vi "MutiType to Enum.vi"(6 "Variant in":variant, 7 "Shift Pressed?":bool, 8 "error in (no error)":errorcluster, 10 "QD Combo Box Ref":refnum<vi>, 11 "QD Launch VI Ref":refnum<vi>) -> (0 "error out":errorcluster, 4 "Variant out":variant)   [LabVIEW 2017, in "String to Enum.lvlib"]
doc: "Converts the selected string, array, ring or combo box into an enum."
uses:
  String to Enum.lvlib
panel:
  in  "Undo Name":string="String to Enum"
  # "Do not change the connector pane of this VI.\n\nSee the block diagram for directions on how to use this template."
  # "Specify the name of the Undo transaction"
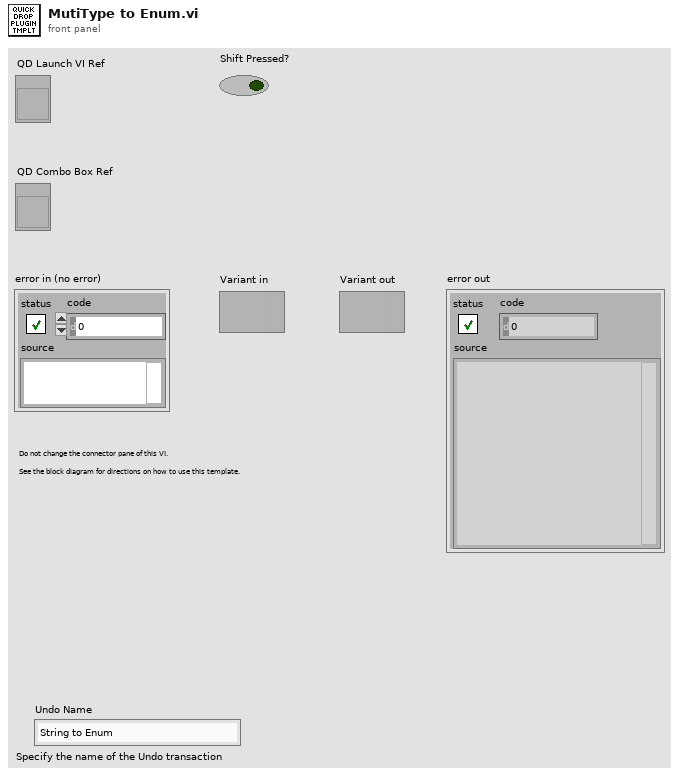
[diagram p1: front panel]
types:
  T1 = typedef "LVPositionTypeDef.ctl" = cluster{"Left":i32, "Top":i32}
  T2 = typedef "LVBoundsTypeDef.ctl" = cluster{"Width":u32, "Height":u32}
  T3 = typedef "LVComboBoxStrsAndValuesArrayTypeDef.ctl" = cluster{"String":string, "Value":string}[]
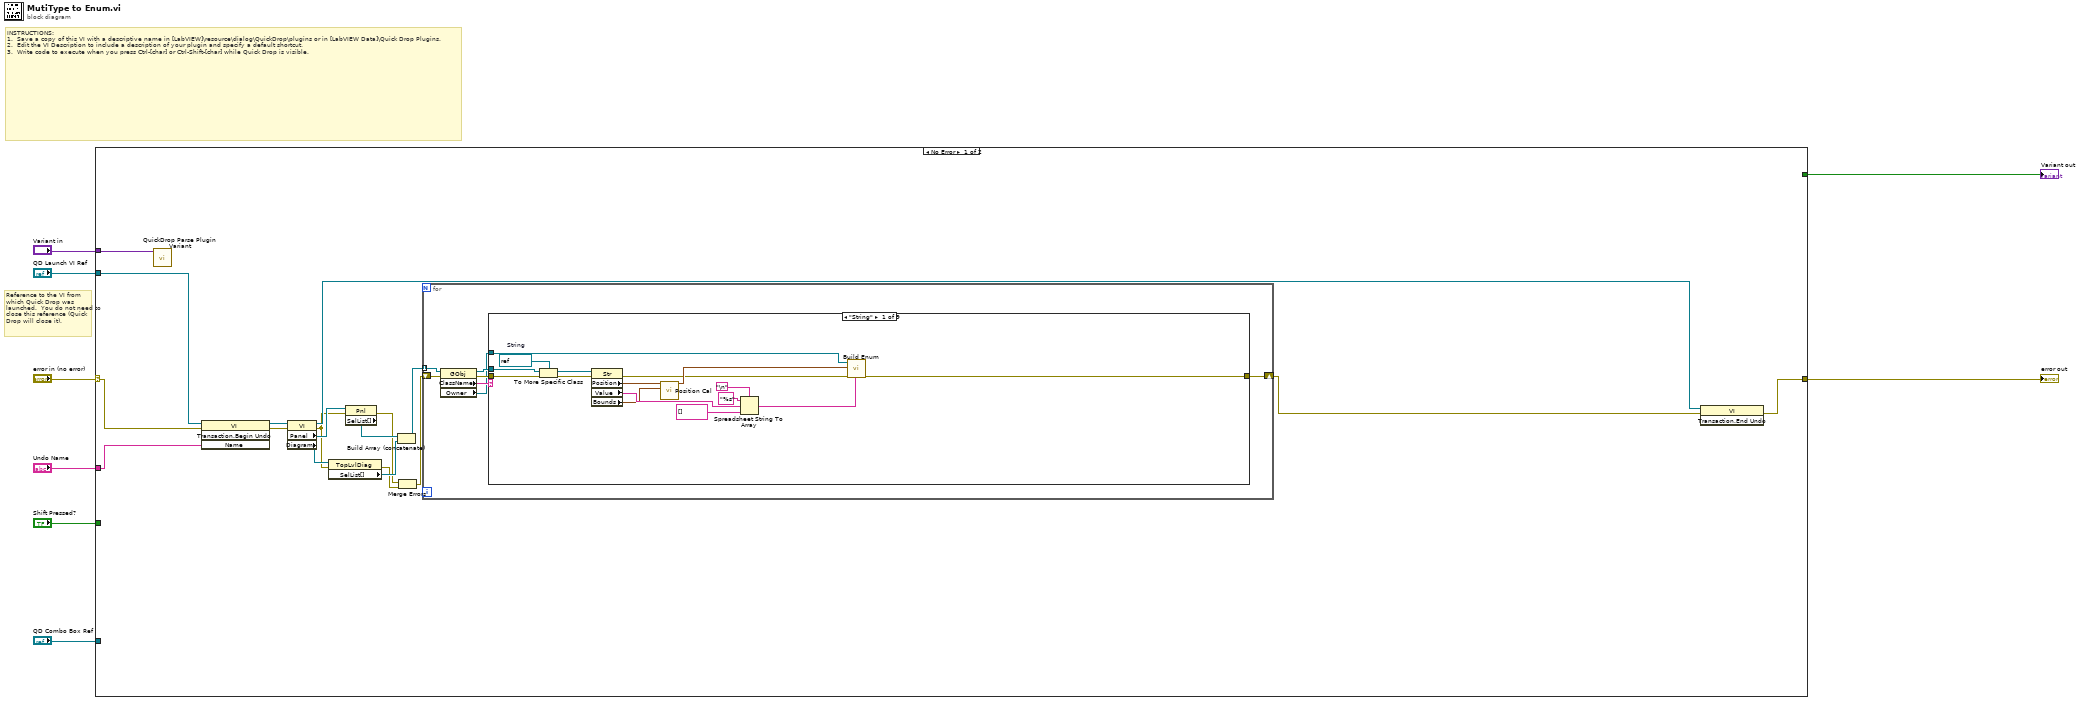
[diagram p0: block diagram]
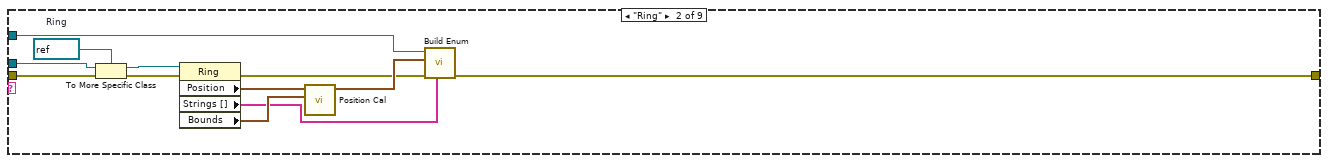
[diagram p2: hidden frame]
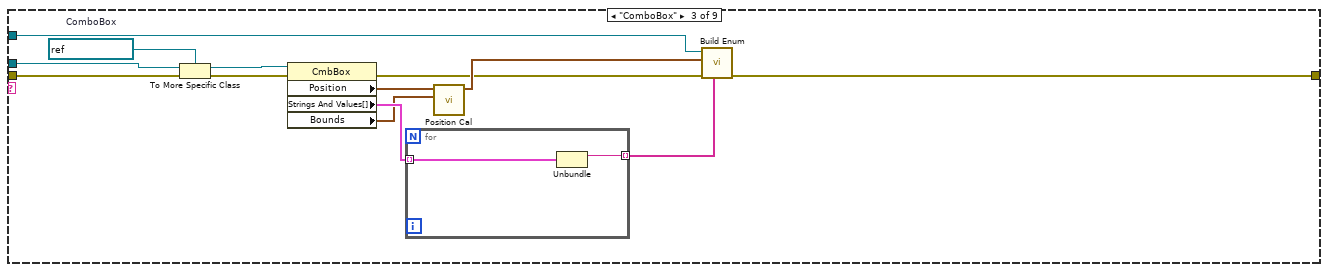
[diagram p3: hidden frame]
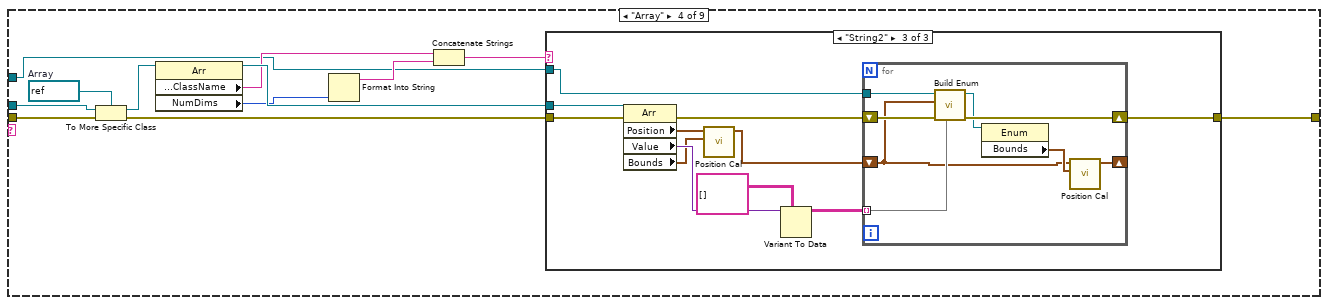
[diagram p4: hidden frame]
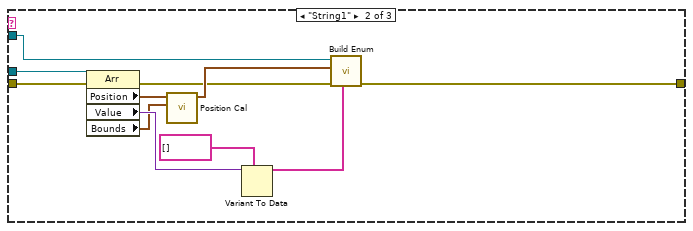
[diagram p6: hidden frame]
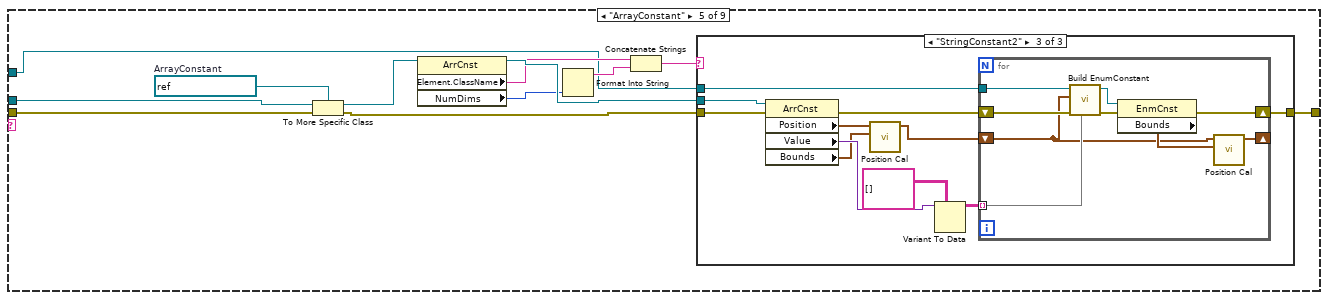
[diagram p7: hidden frame]
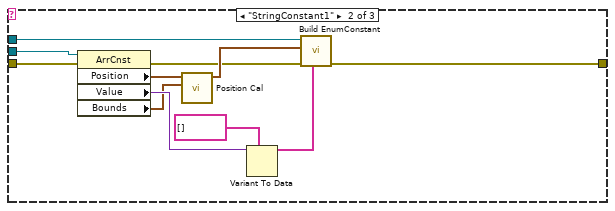
[diagram p9: hidden frame]
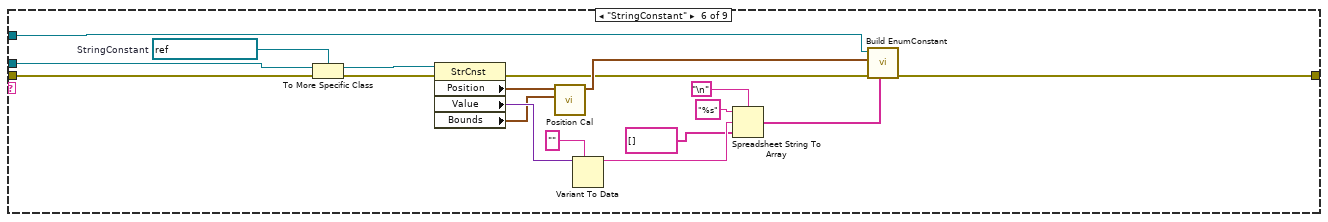
[diagram p10: hidden frame]
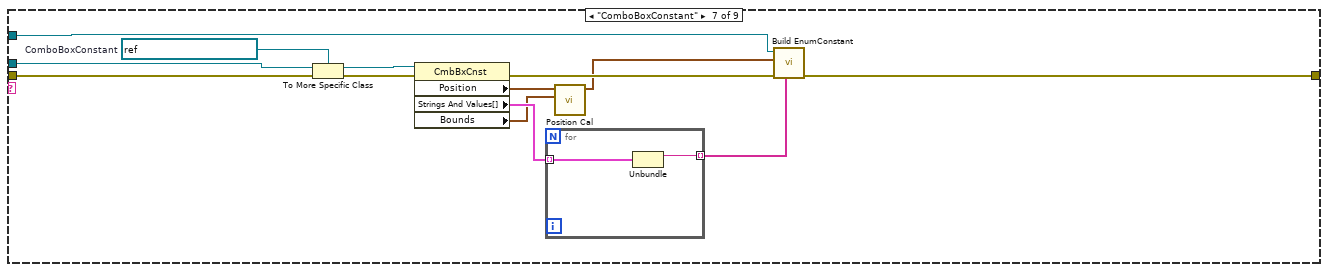
[diagram p11: hidden frame]
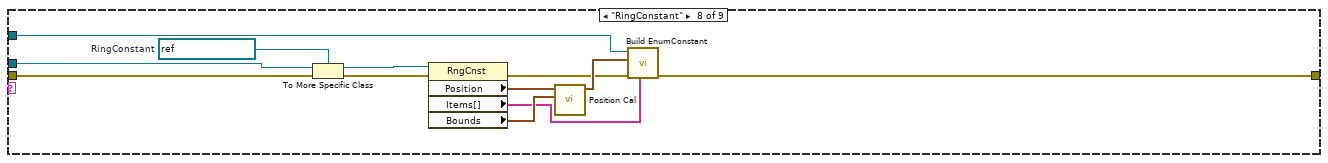
[diagram p12: hidden frame]
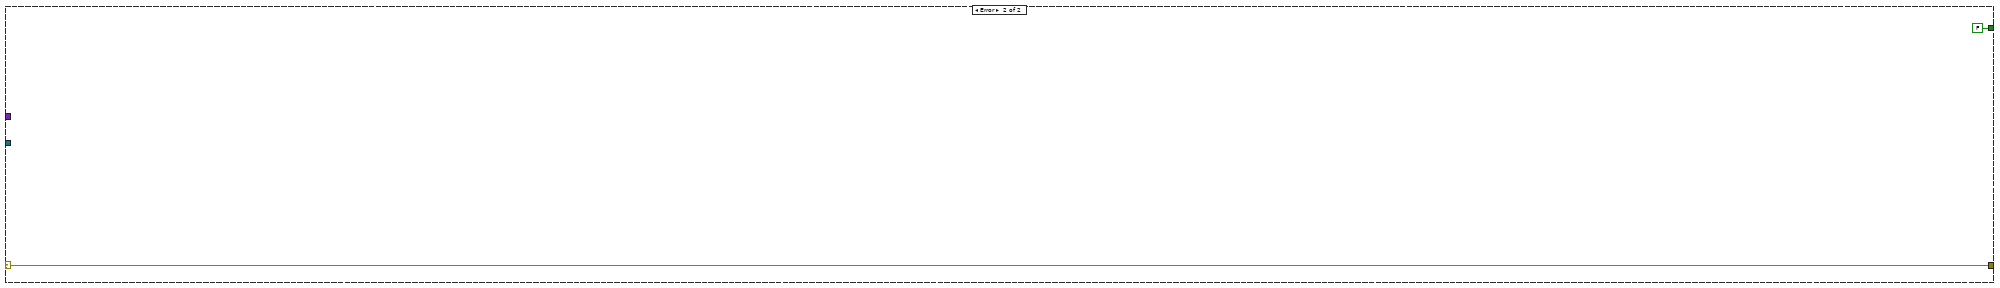
[diagram p14: hidden frame]
diagram:
  # "Reference to the VI from which Quick Drop was launched.  You do not need to close this reference (Quick Drop will close it)."
  # "INSTRUCTIONS:\n1.  Save a copy of this VI with a descriptive name in [LabVIEW]\\resource\\dialog\\QuickDrop\\plugins or in [LabVIEW Data]\\Quick Drop Plugins.\n2.  Edit the VI Description to include a description of your plugin and specify a default shortcut. \n3.  Write code to execute when you press Ctrl-[char] or Ctrl-Shift-[char] while Quick Drop is visible."
  n1 = case shown="No Error" "error in (no error)" {
    selector: "error in (no error)" -> [w23 w211]
    tunnel: [w20 w211] -> w7
    tunnel: "QD Launch VI Ref" -> [w25 _]
    tunnel: "Shift Pressed?" -> [_ _]
    tunnel: "QD Combo Box Ref" -> [_ _]
    tunnel: "Variant in" -> [w18 _]
    tunnel: "Undo Name" -> [w26 _]
    tunnel: [_ FALSE] -> w1
    frame No Error {
      n2 = call <vilib>:"QuickDrop Parse Plugin Variant.vi"("QDKS Variant in"=w18) -> ()  [unwired: 12 in, 3 out]
      n3 = invoke class="VI" method="Transaction.Begin Undo"(reference=w25, error in=w23, "Name"=w26) -> (reference out=w24:refnum<vi>, error out=w22:errorcluster)  [unwired: 1 in, 2 out]
      n4 = property class="VI"(reference=w24, error in=w22) -> (reference out=w21:refnum<vi>, error out=w12:errorcluster, "Panel"=w17:refnum<vi>, "Diagram"=w15:refnum<vi>)
      n5 = property class="TopLvlDiag"(reference=w15, error in=w12) -> (error out=w10:errorcluster, "SelList[]"=w14:refnum<vi>[])  [unwired: 1 out]
      n6 = property class="Pnl"(reference=w17, error in=w12) -> (error out=w11:errorcluster, "SelList[]"=w16:refnum<vi>[])  [unwired: 1 out]
      n7 = Build Array (concatenate)(w16, w14) -> (w13:refnum<vi>[])
      n8 = Merge Errors(w11, w10) -> (w9:errorcluster)
      n9 = for {
        tunnel: w13 -> [w32] mode=indexing
        shift-right: [w33] -> w19
        shift-left: w9 -> [w29]
        n10 = property class="GObj"(reference=w32, error in=w29) -> (reference out=w30:refnum<vi>, error out=w28:errorcluster, "ClassName"=w31:string, "Owner"=w27:refnum<vi>)
        n11 = case shown="\"String\"" w31 {
          tunnel: w27 -> [w40 w56 w65 w77 w120 w168 w187 w199 _]
          tunnel: w30 -> [w49 w61 w74 w88 w131 w181 w194 w208 _]
          tunnel: [w34 w51 w63 w87 w130 w165 w188 w197 w209] -> w33
          tunnel: w28 -> [w44 w58 w71 w85 w128 w174 w190 w205 w209]
          frame "String" {
            w45 = refnum<vi> refnum  # String
            n12 = To More Specific Class(target class=w45, reference=w49, error in=w44) -> (specific class reference=w46:refnum<vi>, error out=w43:errorcluster)
            n13 = property class="Str"(reference=w46, error in=w43) -> (error out=w35:errorcluster, "Position"=w39:T1, "Value"=w42:string, "Bounds"=w38:T2)  [unwired: 1 out]
            n14 = call "Position Cal.vi"("Bounds"=w38, "Position"=w39) -> ("PositionOut"=w37:cluster{u32, "Top":i32})  [unwired: 9 in]
            n15 = Spreadsheet String To Array(delimiter (Tab)="\n", format string="%s", spreadsheet string=w42, array type (2D Dbl)=string[] []) -> (array=w36:string[])
            n16 = call "Build Enum.vi"("Array"=w36, "error in (no error)"=w35, "Position"=w37, "Generic in"=w40) -> ("error out"=w34:errorcluster)  [unwired: 6 in, 1 out]
          }
          frame "Ring" {
            w59 = refnum<vi> refnum  # Ring
            n17 = To More Specific Class(target class=w59, reference=w61, error in=w58) -> (specific class reference=w60:refnum<vi>, error out=w57:errorcluster)
            n18 = property class="Ring"(reference=w60, error in=w57) -> (error out=w50:errorcluster, "Position"=w55:T1, "Strings []"=w52:string[], "Bounds"=w54:T2)  [unwired: 1 out]
            n19 = call "Position Cal.vi"("Bounds"=w54, "Position"=w55) -> ("PositionOut"=w53:cluster{u32, "Top":i32})  [unwired: 9 in]
            n20 = call "Build Enum.vi"("Array"=w52, "error in (no error)"=w50, "Position"=w53, "Generic in"=w56) -> ("error out"=w51:errorcluster)  [unwired: 6 in, 1 out]
          }
          frame "ComboBox" {
            w72 = refnum<vi> refnum  # ComboBox
            n21 = To More Specific Class(target class=w72, reference=w74, error in=w71) -> (specific class reference=w73:refnum<vi>, error out=w70:errorcluster)
            n22 = property class="CmbBox"(reference=w73, error in=w70) -> (error out=w62:errorcluster, "Position"=w68:T1, "Strings And Values[]"=w69:T3, "Bounds"=w67:T2)  [unwired: 1 out]
            n23 = for {
              tunnel: w69 -> [w76] mode=indexing
              tunnel: [w75] -> w64 mode=indexing
              n24 = Unbundle(w76) -> ("String"=w75:string)  [unwired: 1 out]
            }
            n25 = call "Position Cal.vi"("Bounds"=w67, "Position"=w68) -> ("PositionOut"=w66:cluster{u32, "Top":i32})  [unwired: 9 in]
            n26 = call "Build Enum.vi"("Array"=w64, "error in (no error)"=w62, "Position"=w66, "Generic in"=w65) -> ("error out"=w63:errorcluster)  [unwired: 6 in, 1 out]
          }
          frame "Array" {
            w86 = refnum<vi> refnum  # Array
            n27 = To More Specific Class(target class=w86, reference=w88, error in=w85) -> (specific class reference=w83:refnum<vi>, error out=w84:errorcluster)
            n28 = property class="Arr"(reference=w83) -> (reference out=w82:refnum<vi>, "Array Element.ClassName"=w80:string, "NumDims"=w81:u32)  [unwired: 1 in, 1 out]
            n29 = Format Into String(w81) -> (resulting string=w79:string)  [unwired: 3 in, 1 out]
            n30 = Concatenate Strings(w80, w79) -> (w78:string)
            n31 = case shown="\"String2\"" w78 {
              tunnel: [w89 w91 w110] -> w87
              tunnel: w84 -> [w89 w100 w109]
              tunnel: w82 -> [_ w99 w108]
              tunnel: w77 -> [_ w93 w104]
              frame "False", Default {
              }
              frame "String1" {
                n32 = property class="Arr"(reference=w99, error in=w100) -> (error out=w92:errorcluster, "Position"=w95:T1, "Value"=w97:variant, "Bounds"=w94:T2)  [unwired: 1 out]
                n33 = call "Position Cal.vi"("Bounds"=w94, "Position"=w95) -> ("PositionOut"=w96:cluster{u32, "Top":i32})  [unwired: 9 in]
                n34 = Variant To Data(type=string[] [], Variant=w97) -> (data=w90:string[])  [unwired: 1 in, 1 out]
                n35 = call "Build Enum.vi"("Array"=w90, "error in (no error)"=w92, "Position"=w96, "Generic in"=w93) -> ("error out"=w91:errorcluster)  [unwired: 6 in, 1 out]
              }
              frame "String2" {
                n36 = property class="Arr"(reference=w108, error in=w109) -> (error out=w111:errorcluster, "Position"=w103:T1, "Value"=w106:variant, "Bounds"=w102:T2)  [unwired: 1 out]
                n37 = call "Position Cal.vi"("Bounds"=w102, "Position"=w103) -> ("PositionOut"=w101:cluster{u32, "Top":i32})  [unwired: 9 in]
                n38 = Variant To Data(type=string[][] [], Variant=w106) -> (data=w105:string[][])  [unwired: 1 in, 1 out]
                n39 = for {
                  shift-right: [w116] -> w110
                  shift-left: w111 -> [w117]
                  tunnel: w105 -> [w114] mode=indexing
                  tunnel: w104 -> [w118]
                  shift-right: [w119] -> _
                  shift-left: w101 -> [w112]
                  n40 = call "Build Enum.vi"("Array"=w114, "error in (no error)"=w117, "Position"=w112, "Generic in"=w118) -> ("error out"=w116:errorcluster, "EnumRefOut"=w115:refnum<vi>)  [unwired: 6 in]
                  n41 = property class="Enum"(reference=w115) -> ("Bounds"=w113:T2)  [unwired: 1 in, 2 out]
                  n42 = call "Position Cal.vi"("Bounds"=w113, "Position"=w112) -> ("PositionOut"=w119:cluster{u32, "Top":i32})  [unwired: 9 in]
                }
              }
            }
          }
          frame "ArrayConstant" {
            w129 = refnum<vi> refnum  # ArrayConstant
            n43 = To More Specific Class(target class=w129, reference=w131, error in=w128) -> (specific class reference=w126:refnum<vi>, error out=w127:errorcluster)
            n44 = property class="ArrCnst"(reference=w126) -> (reference out=w125:refnum<vi>, "Element.ClassName"=w123:string, "NumDims"=w124:u32)  [unwired: 1 in, 1 out]
            n45 = Format Into String(w124) -> (resulting string=w122:string)  [unwired: 3 in, 1 out]
            n46 = Concatenate Strings(w123, w122) -> (w121:string)
            n47 = case shown="\"StringConstant2\"" w121 {
              tunnel: w120 -> [_ w137 w154]
              tunnel: [w132 w133 w152] -> w130
              tunnel: w127 -> [w132 w143 w151]
              tunnel: w125 -> [_ w142 w150]
              frame "False", Default {
              }
              frame "StringConstant1" {
                n48 = property class="ArrCnst"(reference=w142, error in=w143) -> (error out=w134:errorcluster, "Position"=w139:T1, "Value"=w140:variant, "Bounds"=w138:T2)  [unwired: 1 out]
                n49 = call "Position Cal.vi"("Bounds"=w138, "Position"=w139) -> ("PositionOut"=w136:cluster{u32, "Top":i32})  [unwired: 9 in]
                n50 = Variant To Data(type=string[] [], Variant=w140) -> (data=w135:string[])  [unwired: 1 in, 1 out]
                n51 = call "Build EnumConstant.vi"("Items"=w135, "error in (no error)"=w134, "Position"=w136, "Generic in"=w137) -> ("error out"=w133:errorcluster)  [unwired: 6 in, 1 out]
              }
              frame "StringConstant2" {
                n52 = property class="ArrCnst"(reference=w150, error in=w151) -> (error out=w153:errorcluster, "Position"=w146:T1, "Value"=w148:variant, "Bounds"=w145:T2)  [unwired: 1 out]
                n53 = call "Position Cal.vi"("Bounds"=w145, "Position"=w146) -> ("PositionOut"=w144:cluster{u32, "Top":i32})  [unwired: 9 in]
                n54 = Variant To Data(type=string[][] [], Variant=w148) -> (data=w147:string[][])  [unwired: 1 in, 1 out]
                n55 = for {
                  tunnel: w154 -> [w160]
                  shift-right: [w163] -> w152
                  shift-left: w153 -> [w158]
                  tunnel: w147 -> [w159] mode=indexing
                  shift-right: [w161] -> _
                  shift-left: w144 -> [w155]
                  n56 = call "Build EnumConstant.vi"("Items"=w159, "error in (no error)"=w158, "Position"=w155, "Generic in"=w160) -> ("error out"=w157:errorcluster, "EnumConstantRef"=w156:refnum<vi>)  [unwired: 6 in]
                  n57 = property class="EnmCnst"(reference=w156, error in=w157) -> (error out=w163:errorcluster, "Bounds"=w162:T2)  [unwired: 1 out]
                  n58 = call "Position Cal.vi"("Bounds"=w162, "Position"=w155) -> ("PositionOut"=w161:cluster{u32, "Top":i32})  [unwired: 9 in]
                }
              }
            }
          }
          frame "StringConstant" {
            w175 = refnum<vi> refnum  # StringConstant
            n59 = To More Specific Class(target class=w175, reference=w181, error in=w174) -> (specific class reference=w176:refnum<vi>, error out=w173:errorcluster)
            n60 = property class="StrCnst"(reference=w176, error in=w173) -> (error out=w166:errorcluster, "Position"=w170:T1, "Value"=w172:variant, "Bounds"=w169:T2)  [unwired: 1 out]
            n61 = call "Position Cal.vi"("Bounds"=w169, "Position"=w170) -> ("PositionOut"=w167:cluster{u32, "Top":i32})  [unwired: 9 in]
            n62 = Variant To Data(type="", Variant=w172) -> (data=w178:string)  [unwired: 1 in, 1 out]
            n63 = Spreadsheet String To Array(delimiter (Tab)="\n", format string="%s", spreadsheet string=w178, array type (2D Dbl)=string[] []) -> (array=w164:string[])
            n64 = call "Build EnumConstant.vi"("Items"=w164, "error in (no error)"=w166, "Position"=w167, "Generic in"=w168) -> ("error out"=w165:errorcluster)  [unwired: 6 in, 1 out]
          }
          frame "ComboBoxConstant" {
            w191 = refnum<vi> refnum  # ComboBoxConstant
            n65 = To More Specific Class(target class=w191, reference=w194, error in=w190) -> (specific class reference=w192:refnum<vi>, error out=w189:errorcluster)
            n66 = property class="CmbBxCnst"(reference=w192, error in=w189) -> (error out=w193:errorcluster, "Position"=w184:T1, "Strings And Values[]"=w186:T3, "Bounds"=w183:T2)  [unwired: 1 out]
            n67 = for {
              tunnel: w186 -> [w196] mode=indexing
              tunnel: [w195] -> w185 mode=indexing
              n68 = Unbundle(w196) -> ("String"=w195:string)  [unwired: 1 out]
            }
            n69 = call "Position Cal.vi"("Bounds"=w183, "Position"=w184) -> ("PositionOut"=w182:cluster{u32, "Top":i32})  [unwired: 9 in]
            n70 = call "Build EnumConstant.vi"("Items"=w185, "error in (no error)"=w193, "Position"=w182, "Generic in"=w187) -> ("error out"=w188:errorcluster)  [unwired: 6 in, 1 out]
          }
          frame "RingConstant" {
            w206 = refnum<vi> refnum  # RingConstant
            n71 = To More Specific Class(target class=w206, reference=w208, error in=w205) -> (specific class reference=w207:refnum<vi>, error out=w204:errorcluster)
            n72 = property class="RngCnst"(reference=w207, error in=w204) -> (error out=w198:errorcluster, "Position"=w202:T1, "Items[]"=w200:string[], "Bounds"=w201:T2)  [unwired: 1 out]
            n73 = call "Position Cal.vi"("Bounds"=w201, "Position"=w202) -> ("PositionOut"=w203:cluster{u32, "Top":i32})  [unwired: 9 in]
            n74 = call "Build EnumConstant.vi"("Items"=w200, "error in (no error)"=w198, "Position"=w203, "Generic in"=w199) -> ("error out"=w197:errorcluster)  [unwired: 6 in, 1 out]
          }
          frame "Error", Default {
          }
        }
      }
      n75 = invoke class="VI" method="Transaction.End Undo"(reference=w21, error in=w19) -> (error out=w20:errorcluster)  [unwired: 1 in, 2 out]
    }
    frame Error {
    }
  }
  "error out" <- w7
  "Variant out" <- w1
